vi "IO Docs.vi"(0 "Analog IO":dbl[](array[numeric]), 2 "BIAS DIFF":T3 {"DIFF" step=10.0; "BIAS" step=10.0}, 3 "Digital IO":bool[](array[boolean]), 4 "GXVALS Input":T1 {"g2rdggain" step=1e-05; "g2rdgoffset" step=1e-05; "g2spgain" step=1e-05; "g2spoffset" step=1e-05; "g1rdggain" step=1e-05; "g1rdgoffset" step=1e-05; "g1spgain" step=1e-05; "g1spoffset" step=1e-05}, 5 "Error In":errorcluster, 8 "User Creds":T2, 9 "OffsetGain":dbl[](array[numeric])) -> (10 "OffsetGain Out":dbl[](array[numeric]), 11 "BIAS DIFF Out":T3 {"DIFF" step=10.0; "BIAS" step=10.0}, 14 "Analog IO Out":dbl[](array[numeric]), 17 "GXVALS Output":T1 {"g2rdggain" step=1e-05; "g2rdgoffset" step=1e-05; "g2spgain" step=1e-05; "g2spoffset" step=1e-05; "g1rdggain" step=1e-05; "g1rdgoffset" step=1e-05; "g1spgain" step=1e-05; "g1spoffset" step=1e-05}, 19 "Error Out":errorcluster)   [LabVIEW 2023, in "QSM - IODocs.lvlib"]
uses:
  QSM - IODocs.lvlib
  Controls/AnalogIOAll.ctl
  Controls/AnalogIOsingle.ctl
  QSM - Main/Controls/biasdiff.ctl
  QSM - Main/Controls/gridvals.ctl
  UserCredentials.ctl
  Controls/State Machine Message.ctl
  Controls/Message Queue Element Position.ctl
  <vilib>/event_ctls.llb/usereventprio.ctl
  Controls/Event Handler Message.ctl
  QSM - Main/QSM - Main.lvlib
panel:
  in  "CLOSE":bool
  in  "GXVALS":T1 {"g2rdggain" step=1e-05; "g2rdgoffset" step=1e-05; "g2spgain" step=1e-05; "g2spoffset" step=1e-05; "g1rdggain" step=1e-05; "g1rdgoffset" step=1e-05; "g1spgain" step=1e-05; "g1spoffset" step=1e-05}
  out "DIO Cluster":T4
  in  "Analog IO Cluster":T5 {"AIO Cluster remIfrdg"."IOspgain" step=1e-05; "AIO Cluster remIfrdg"."IOspoffset" step=1e-05; "AIO Cluster remEfDrRdg"."IOspgain" step=1e-05; "AIO Cluster remEfDrRdg"."IOspoffset" step=1e-05; "AIO Cluster remEfDrSP"."IOspgain" step=1e-05; "AIO Cluster remEfDrSP"."IOspoffset" step=1e-05; "AIO Cluster remMArdg"."IOspgain" step=1e-05; "AIO Cluster remMArdg"."IOspoffset" step=1e-05; "AIO Cluster remMASP"."IOspgain" step=1e-05; "AIO Cluster remMASP"."IOspoffset" step=1e-05; "AIO Cluster remKVrdg"."IOspgain" step=1e-05; "AIO Cluster remKVrdg"."IOspoffset" step=1e-05; "AIO Cluster remKVSP"."IOspgain" step=1e-05; "AIO Cluster remKVSP"."IOspoffset" step=1e-05}
  # "ANALOG I/O"
  # "GRID TANK VALUES"
  # "DIGITAL I/O"
  # "OFFSET"
  # "OFFSET"
  # "GAIN"
  # "GAIN"
  # "OFFSET"
  # "OFFSET"
  # "GAIN"
  # "GAIN"
  # "OFFSET"
  # "OFFSET"
  # "GAIN"
  # "GAIN"
  # "OFFSET"
  # "OFFSET"
  # "GAIN"
  # "GAIN"
  # "OFFSET"
  # "OFFSET"
  # "GAIN"
  # "GAIN"
  # "OFFSET"
  # "OFFSET"
  # "GAIN"
  # "GAIN"
  # "remKVSP"
  # "remKVrdg"
  # "remMASP"
  # "remMArdg"
  # "remEfDrSP"
  # "remEfDrRdg"
  # "remIfrdg"
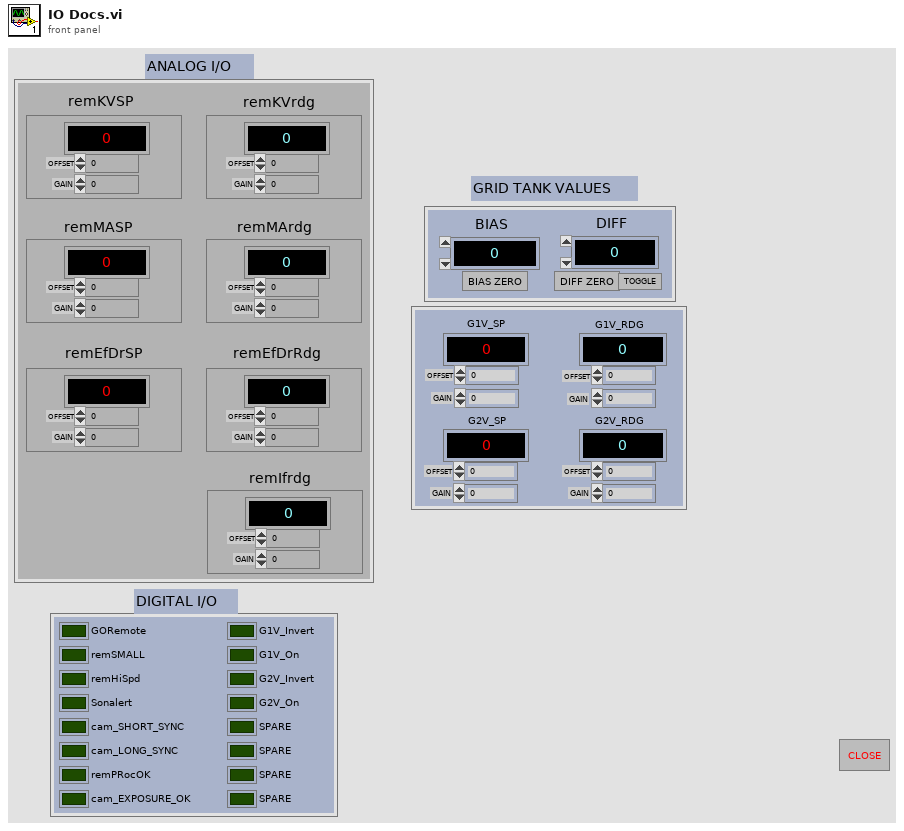
[diagram p1: front panel]
types:
  T1 = typedef "QSM - Main.lvlib/gridvals.ctl" = cluster{"G1V_SP":dbl, "G2V_SP":dbl, "G1V_RDG":dbl, "G2V_RDG":dbl, "g1spoffset":dbl, "g1spgain":dbl, "g1rdgoffset":dbl, "g1rdggain":dbl, "g2spoffset":dbl, "g2spgain":dbl, "g2rdgoffset":dbl, "g2rdggain":dbl}
  T2 = typedef "UserCredentials.ctl" = cluster{"Badge Number":string, "Name":string, "Access":enum16{"", "Operator", "Admin", "Engineer"}}
  T3 = typedef "QSM - Main.lvlib/biasdiff.ctl" = cluster{"BIAS":dbl, "BIAS_ZER":bool, "DIFF_ZER":bool, "DIFF_TOGGLE":bool, "DIFF":dbl}
  T4 = cluster{"GORemote":bool, "remSMALL":bool, "remHiSpd":bool, "Sonalert":bool, "cam_SHORT_SYNC":bool, "cam_LONG_SYNC":bool, "remPRocOK":bool, "cam_EXPOSURE_OK":bool, "G1V_Invert":bool, "G1V_On":bool, "G2V_Invert":bool, "G2V_On":bool, "SPARE":bool, "SPARE":bool, "SPARE":bool, "SPARE":bool}
  T5 = typedef "QSM - IODocs.lvlib/AnalogIOAll.ctl" = cluster{"AIO Cluster remKVSP":T6, "AIO Cluster remKVrdg":T6, "AIO Cluster remMASP":T6, "AIO Cluster remMArdg":T6, "AIO Cluster remEfDrSP":T6, "AIO Cluster remEfDrRdg":T6, "AIO Cluster remIfrdg":T6}
  T6 = typedef "QSM - IODocs.lvlib/AnalogIOsingle.ctl" = cluster{"I/O":dbl, "IOspoffset":dbl, "IOspgain":dbl}
  T7 = typedef "QSM - IODocs.lvlib/State Machine Message.ctl" = enum16{"Initialize", "BIAS ZERO", "DIFF ZERO", "DIFF TOGGLE", "UpdateAIO", "UpdateBiasDiff", "GxValsUpdate", "OffsetGainUpdate", "APIAIOUpdate", "APIGridValsUpdate", "APIBiasDiffUpdate", "Handle Error", "Exit"}
  T8 = typedef "QSM - IODocs.lvlib/User Event Reference.ctl" = refnum<user-event>
  T9 = typedef "QSM - IODocs.lvlib/User Event Registration Reference.ctl" = refnum<event-registration>
  T10 = typedef "QSM - IODocs.lvlib/Event Handler Message.ctl" = enum16{"Exit"}
  T11 = typedef "usereventprio.ctl" = enum32{"high priority", "normal priority"}
  T12 = cluster{"Value[0]":bool, "Value[1]":bool, "Value[2]":bool, "Value[3]":bool, "Value[4]":bool, "Value[5]":bool, "Value[6]":bool, "Value[7]":bool, "Value[8]":bool, "Value[9]":bool, "Value[10]":bool, "Value[11]":bool, "Value[12]":bool, "Value[13]":bool, "Value[14]":bool, "Value[15]":bool}
  T13 = cluster{"Value[0]":dbl, "Value[1]":dbl, "Value[2]":dbl, "Value[3]":dbl, "Value[4]":dbl, "Value[5]":dbl, "Value[6]":dbl, "Value[7]":dbl, "Value[8]":dbl, "Value[9]":dbl, "Value[10]":dbl, "Value[11]":dbl, "Value[12]":dbl, "Value[13]":dbl, "Value[14]":dbl, "Value[15]":dbl, "Value[16]":dbl, "Value[17]":dbl, "Value[18]":dbl, "Value[19]":dbl, "Value[20]":dbl, "Value[21]":dbl}
  T14 = enum8{"Enabled", "Disabled", "Disabled and Grayed Out"}
  T15 = cluster{"Value[0]":dbl, "Value[1]":dbl, "Value[2]":dbl, "Value[3]":dbl, "Value[4]":dbl, "Value[5]":dbl, "Value[6]":dbl, "Value[7]":dbl, "Value[8]":dbl, "Value[9]":dbl, "Value[10]":dbl}
  T16 = cluster{"Analog IO[0]":dbl, "Analog IO[1]":dbl, "Analog IO[2]":dbl, "Analog IO[3]":dbl, "Analog IO[4]":dbl, "Analog IO[5]":dbl, "Analog IO[6]":dbl, "Analog IO[7]":dbl, "Analog IO[8]":dbl, "Analog IO[9]":dbl, "Analog IO[10]":dbl}
  T17 = typedef "QSM - IODocs.lvlib/Message Queue Element Position.ctl" = enum16{"Front", "Back"}
  T18 = typedef "QMH - Library.lvlib/Event Handler Message.ctl" = enum16{"Exit"}
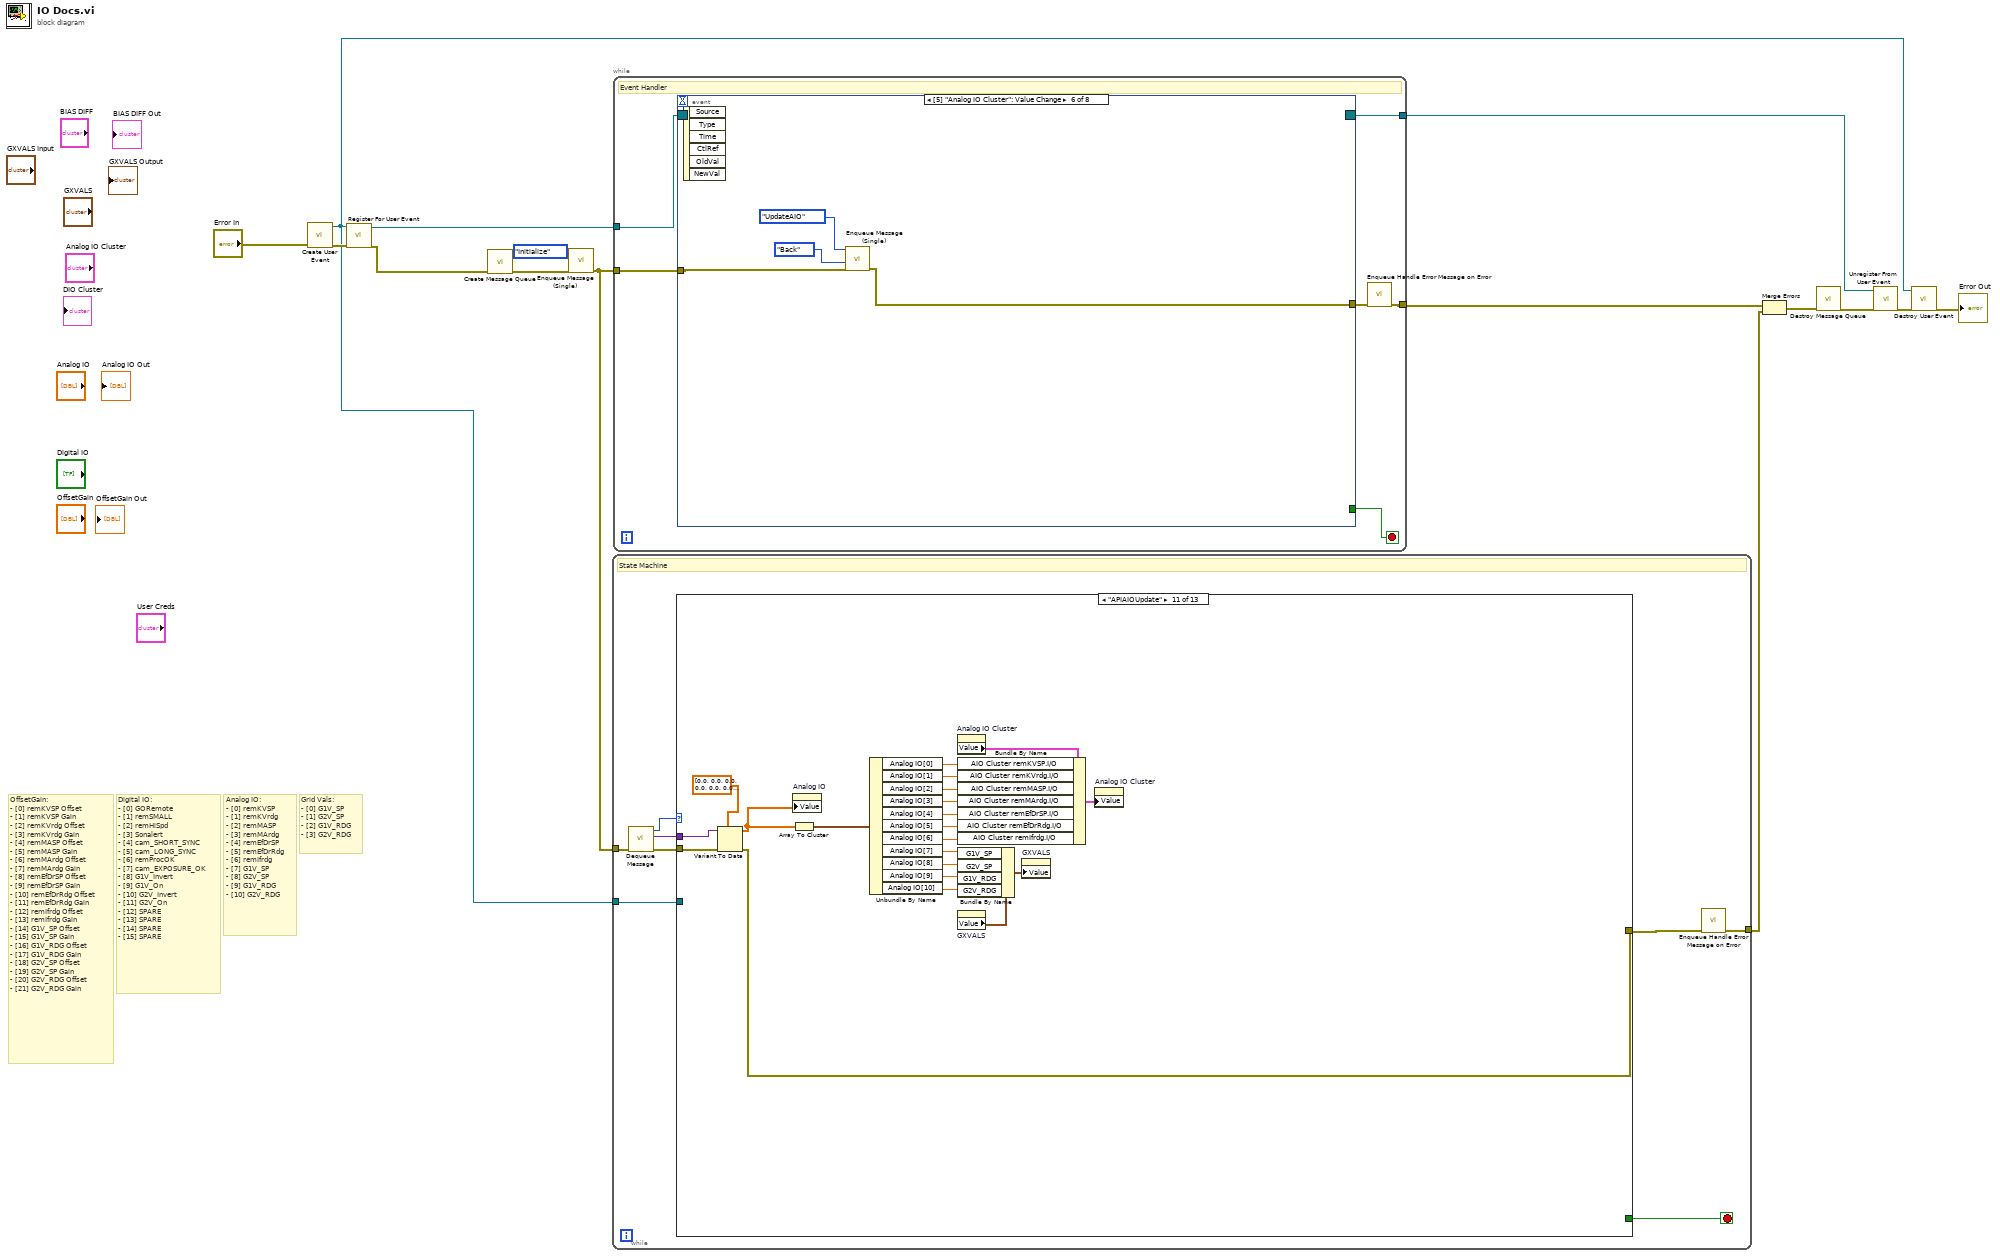
[diagram p0: block diagram]
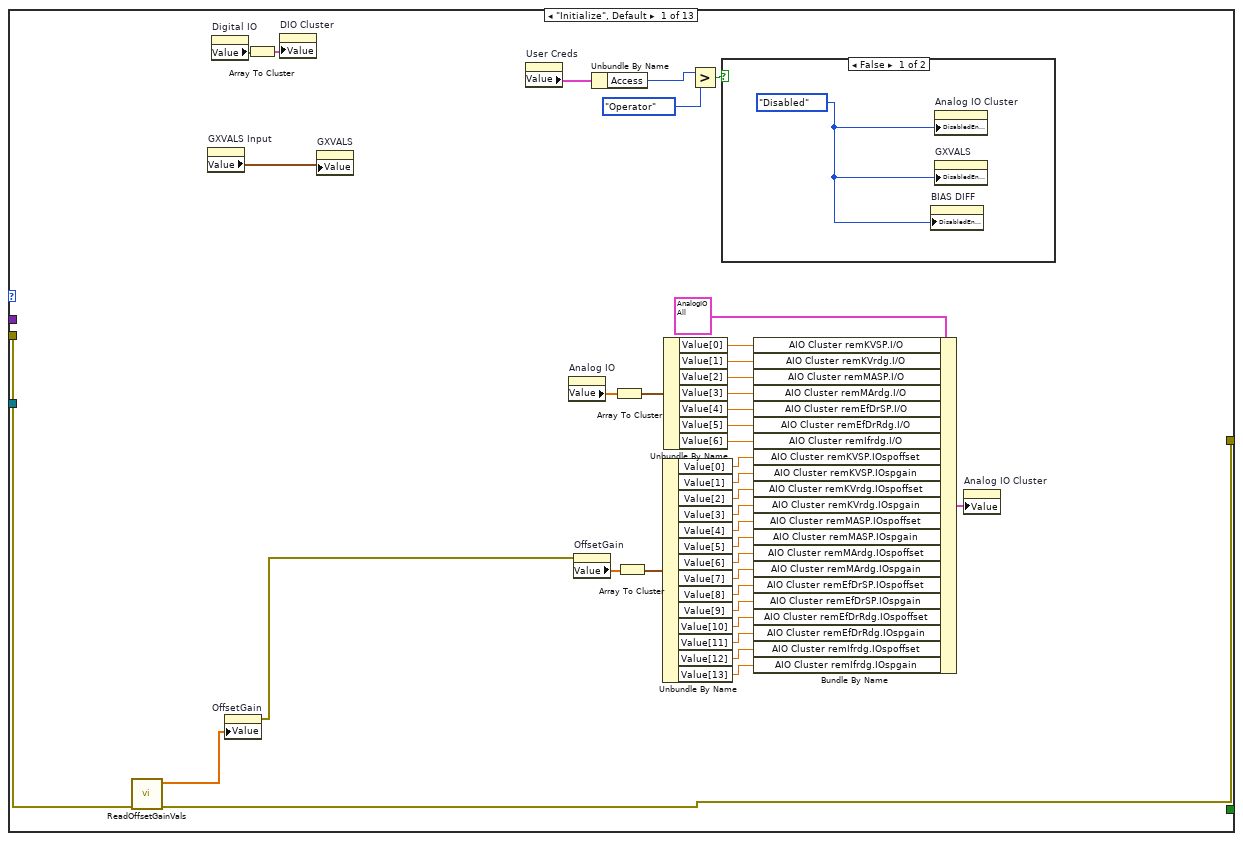
[diagram p2: hidden frame]
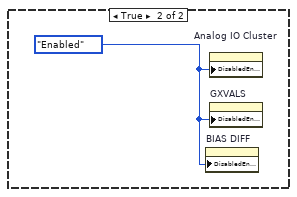
[diagram p3: hidden frame]
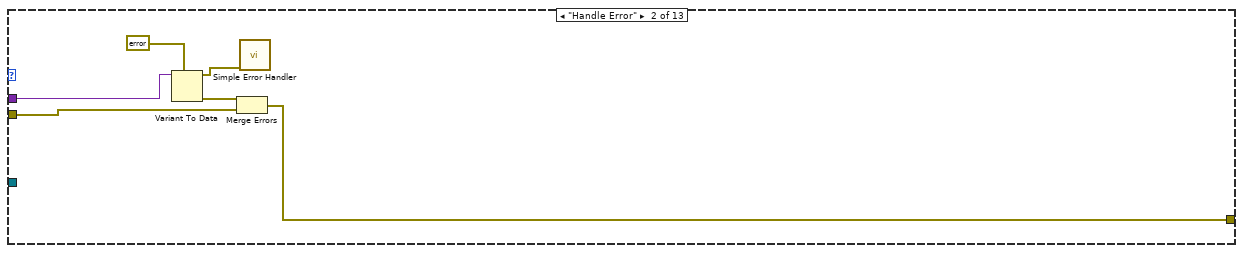
[diagram p4: hidden frame]
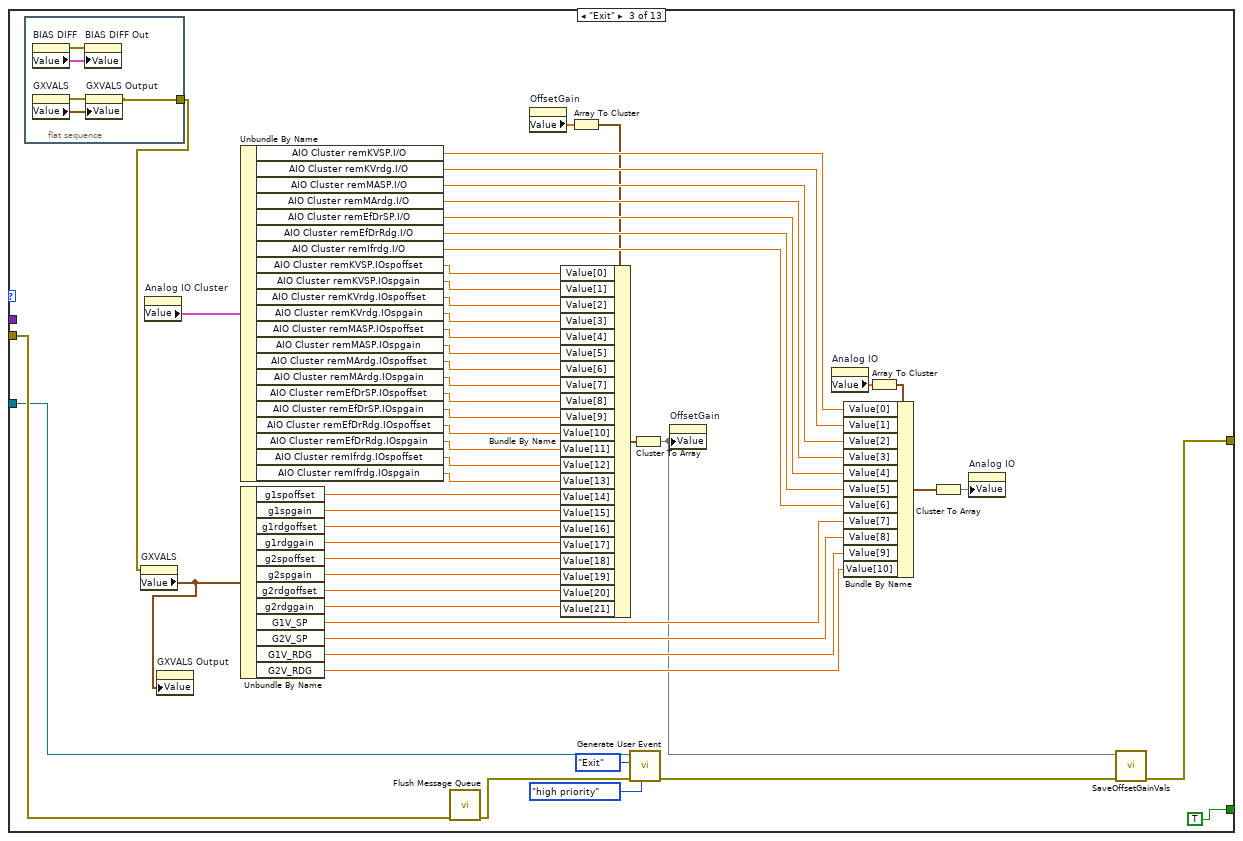
[diagram p5: hidden frame]
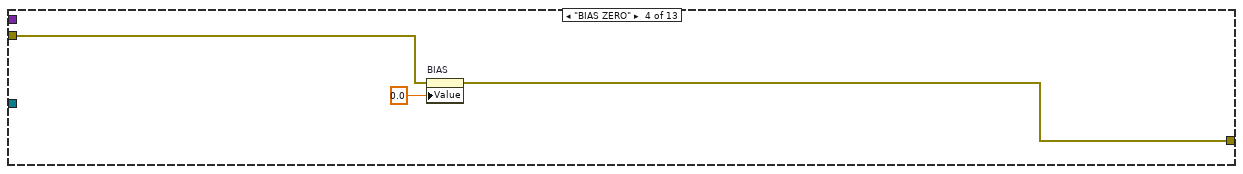
[diagram p6: hidden frame]
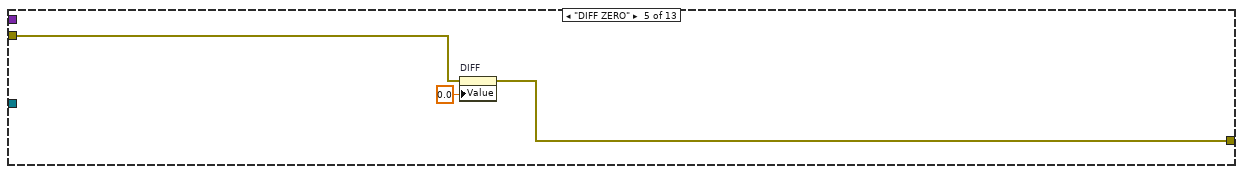
[diagram p7: hidden frame]
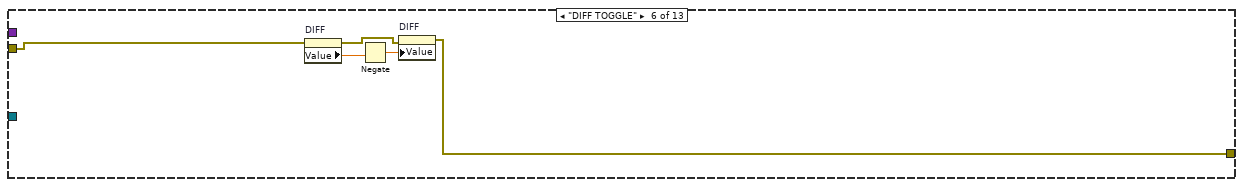
[diagram p8: hidden frame]
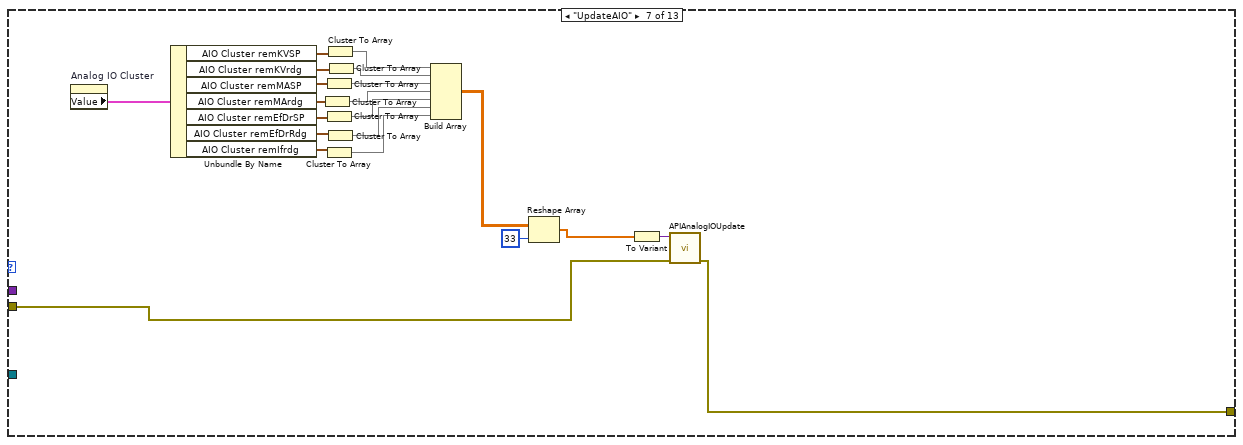
[diagram p9: hidden frame]
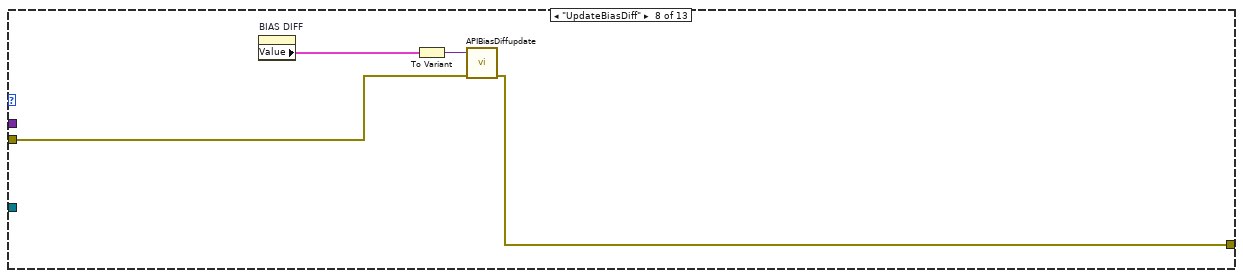
[diagram p10: hidden frame]
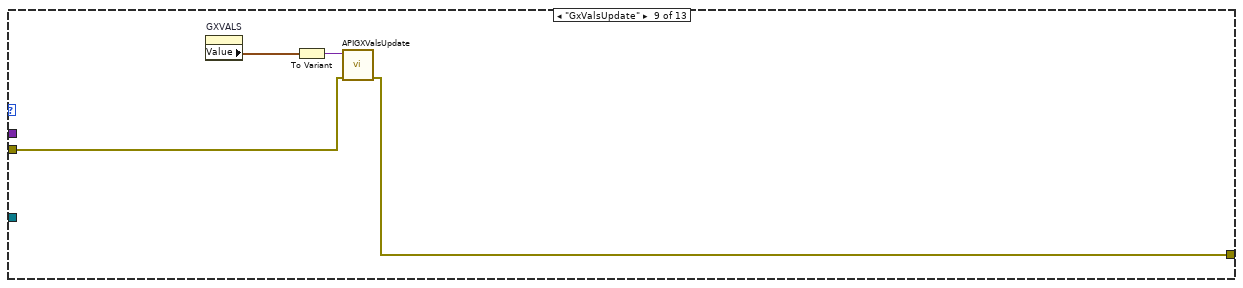
[diagram p11: hidden frame]
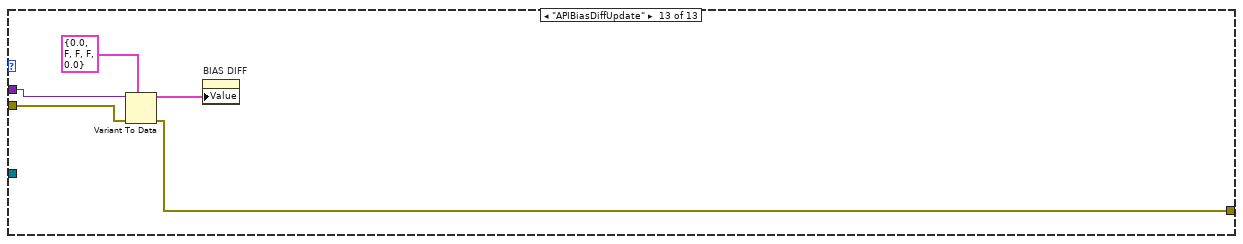
[diagram p14: hidden frame]
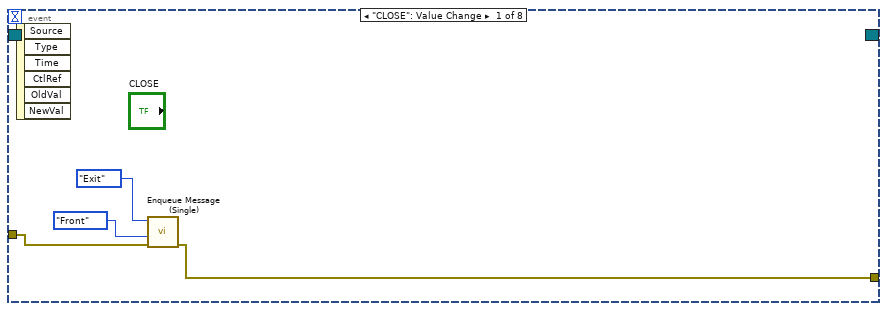
[diagram p15: hidden frame]
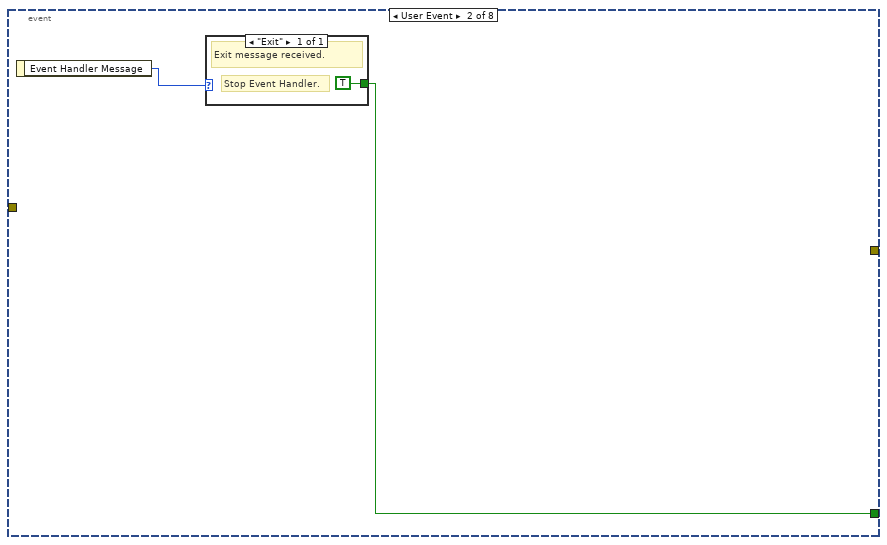
[diagram p16: hidden frame]
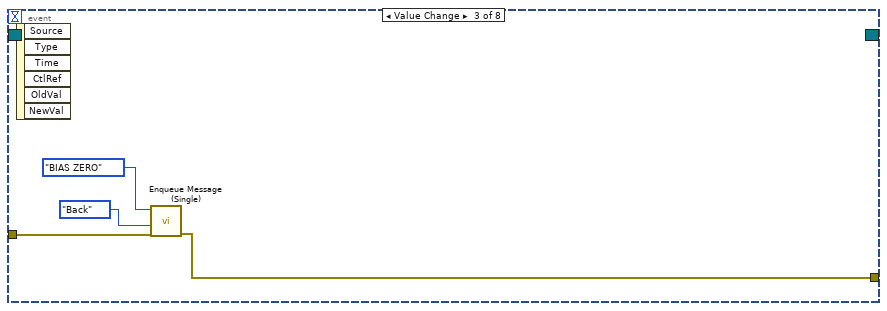
[diagram p17: hidden frame]
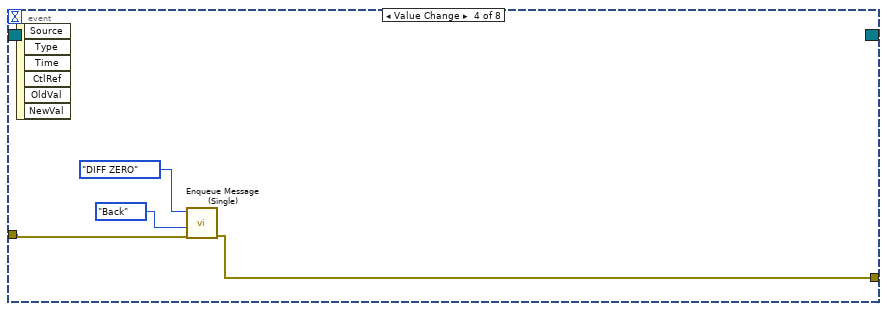
[diagram p18: hidden frame]
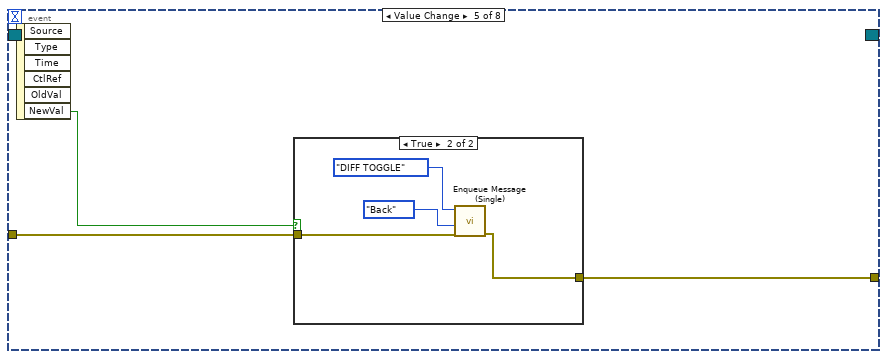
[diagram p19: hidden frame]
diagram:
  # "OffsetGain:\n- [0] remKVSP Offset\n- [1] remKVSP Gain\n- [2] remKVrdg Offset\n- [3] remKVrdg Gain\n- [4] remMASP Offset\n- [5] remMASP Gain\n- [6] remMArdg Offset\n- [7] remMArdg Gain\n- [8] remEfDrSP Offset\n- [9] remEfDrSP Gain\n- [10] remEfDrRdg Offset\n- [11] remEfDrRdg Gain\n- [12] remIfrdg Offset\n- [13] remIfrdg Gain\n- [14] G1V_SP Offset\n- [15] G1V_SP Gain\n- [16] G1V_RDG Offset\n- [17] G1V_RDG Gain\n- [18] G2V_SP Offset\n- [19] G2V_SP Gain\n- [20] G2V_RDG Offset\n- [21] G2V_RDG Gain"
  # "Digital IO:\n- [0] GORemote\n- [1] remSMALL\n- [2] remHiSpd\n- [3] Sonalert\n- [4] cam_SHORT_SYNC\n- [5] cam_LONG_SYNC\n- [6] remProcOK\n- [7] cam_EXPOSURE_OK\n- [8] G1V_Invert\n- [9] G1V_On\n- [10] G2V_Invert\n- [11] G2V_On\n- [12] SPARE\n- [13] SPARE\n- [14] SPARE\n- [15] SPARE"
  # "Grid Vals:\n- [0] G1V_SP\n- [1] G2V_SP\n- [2] G1V_RDG\n- [3] G2V_RDG"
  # "Analog IO:\n- [0] remKVSP\n- [1] remKVrdg\n- [2] remMASP\n- [3] remMArdg\n- [4] remEfDrSP\n- [5] remEfDrRdg\n- [6] remIfrdg\n- [7] G1V_SP\n- [8] G2V_SP\n- [9] G1V_RDG\n- [10] G2V_RDG"
  n1 = call "Create User Event.vi"("Error In"="Error In") -> ("Error Out"=w8:errorcluster, "User Event Reference"=w1:T8)  [unwired: 9 in]
  n2 = call "Register For User Event.vi"("Error In"=w8, "User Event Reference"=w1) -> ("Error Out"=w7:errorcluster, "User Event Registration Reference"=w6:T9)  [unwired: 8 in]
  n3 = call "Create Message Queue.vi"("Error In"=w7) -> ("Error Out"=w15:errorcluster)  [unwired: 10 in]
  n4 = call "Enqueue Message (Single).vi"("Error In"=w15, "State Machine Message"=State_Machine_Message."Initialize") -> ("Error Out"=w10:errorcluster)  [unwired: 9 in]
  n5 = while {
    tunnel: [w22] -> w13
    tunnel: w10 -> [w17]
    tunnel: w1 -> [w16]
    stop <- w23 stop-if-true
    # "State Machine"
    n6 = call "Dequeue Message.vi"("Error In"=w17) -> ("Error Out"=w21:errorcluster, "Data"=w19:variant, "State Machine Message"=w20:T7)  [unwired: 8 in]
    n7 = case shown="\"APIAIOUpdate\"" w20 {
      tunnel: [_ _ TRUE _ _ _ _ _ _ _ _ _ _] -> w23
      tunnel: w21 -> [w27 w66 w121 w127 w130 w136 w157 w161 w165 w167 w187 w189 w192]
      tunnel: w19 -> [_ w65 _ _ _ _ _ _ _ _ w188 _ w194]
      tunnel: [w26 w64 w71 w129 w132 w133 w156 w160 w164 w167 w186 w189 w191] -> w18
      tunnel: w16 -> [_ _ w73 _ _ _ _ _ _ _ _ _ _]
      frame "Initialize", Default {
        n8 = call "ReadOffsetGainVals.vi"("error in"=w27) -> ("error out"=w26:errorcluster, "Array"=w25:dbl[])  [unwired: 9 in]
        n9 = property on="GXVALS Input" class="Clust (strict)"() -> ("Value"=w28:T1)  [unwired: 2 in, 2 out]
        n10 = property on="Digital IO" class="Arr (strict)"() -> ("Value"=w58:bool[])  [unwired: 2 in, 2 out]
        n11 = property on="OffsetGain" class="Arr (strict)"("Value"=w25) -> (error out=w24:errorcluster)  [unwired: 2 in, 1 out]
        n12 = Array To Cluster(array=w58) -> (cluster=w57:T12)
        n13 = property on="DIO Cluster" class="Clust (strict)"("Value"=w57) -> ()  [unwired: 2 in, 2 out]
        n14 = property on="GXVALS" class="Clust (strict)"("Value"=w28) -> ()  [unwired: 2 in, 2 out]
        n15 = property on="User Creds" class="Clust (strict)"() -> ("Value"=w31:T2)  [unwired: 2 in, 2 out]
        n16 = property on="Analog IO" class="Arr (strict)"() -> ("Value"=w61:dbl[])  [unwired: 2 in, 2 out]
        n17 = property on="OffsetGain" class="Arr (strict)"(error in=w24) -> ("Value"=w49:dbl[])  [unwired: 1 in, 2 out]
        n18 = Unbundle By Name(w31) -> ("Access"=w30:enum16{"", "Operator", "Admin", "Engineer"})
        n19 = Array To Cluster(array=w61) -> (cluster=w33:T13)
        n20 = Array To Cluster(array=w49) -> (cluster=w48:T13)
        n21 = Unbundle By Name(w48) -> ("Value[0]"=w47:dbl, "Value[1]"=w46:dbl, "Value[2]"=w45:dbl, "Value[3]"=w44:dbl, "Value[4]"=w43:dbl, "Value[5]"=w42:dbl, "Value[6]"=w41:dbl, "Value[7]"=w40:dbl, "Value[8]"=w39:dbl, "Value[9]"=w38:dbl, "Value[10]"=w37:dbl, "Value[11]"=w36:dbl, "Value[12]"=w35:dbl, "Value[13]"=w34:dbl)
        n22 = Unbundle By Name(w33) -> ("Value[0]"=w56:dbl, "Value[1]"=w55:dbl, "Value[2]"=w54:dbl, "Value[3]"=w53:dbl, "Value[4]"=w52:dbl, "Value[5]"=w51:dbl, "Value[6]"=w50:dbl)
        n23 = Greater?(x=w30, y=enum16{"", "Operator", "Admin", "Engineer"}."Operator") -> (0:w32:bool)
        n24 = case shown="False" w32 {
          frame False {
            w62 = T14."Disabled" ("Disabled")
            n25 = property on="BIAS DIFF" class="Clust (strict)"("DisabledEnum"=w62) -> ()  [unwired: 2 in, 2 out]
            n26 = property on="Analog IO Cluster" class="Clust (strict)"("DisabledEnum"=w62) -> ()  [unwired: 2 in, 2 out]
            n27 = property on="GXVALS" class="Clust (strict)"("DisabledEnum"=w62) -> ()  [unwired: 2 in, 2 out]
          }
          frame True {
            w63 = T14."Enabled" ("Disabled")
            n28 = property on="BIAS DIFF" class="Clust (strict)"("DisabledEnum"=w63) -> ()  [unwired: 2 in, 2 out]
            n29 = property on="Analog IO Cluster" class="Clust (strict)"("DisabledEnum"=w63) -> ()  [unwired: 2 in, 2 out]
            n30 = property on="GXVALS" class="Clust (strict)"("DisabledEnum"=w63) -> ()  [unwired: 2 in, 2 out]
          }
        }
        n31 = Bundle By Name(cluster=T5 {"AIO Cluster remKVSP"={"I/O"=0.0, "IOspoffset"=0.0, "IOspgain"=0.0}, "AIO Cluster remKVrdg"={"I/O"=0.0, "IOspoffset"=0.0, "IOspgain"=0.0}, "AIO Cluster remMASP"={"I/O"=0.0, "IOspoffset"=0.0, "IOspgain"=0.0}, "AIO Cluster remMArdg"={"I/O"=0.0, "IOspoffset"=0.0, "IOspgain"=0.0}, "AIO Cluster remEfDrSP"={"I/O"=0.0, "IOspoffset"=0.0, "IOspgain"=0.0}, "AIO Cluster remEfDrRdg"={"I/O"=0.0, "IOspoffset"=0.0, "IOspgain"=0.0}, "AIO Cluster remIfrdg"={"I/O"=0.0, "IOspoffset"=0.0, "IOspgain"=0.0}} ("Analog IO Cluster"), "AIO Cluster remKVSP.I/O"=w56, "AIO Cluster remKVrdg.I/O"=w55, "AIO Cluster remMASP.I/O"=w54, "AIO Cluster remMArdg.I/O"=w53, "AIO Cluster remEfDrSP.I/O"=w52, "AIO Cluster remEfDrRdg.I/O"=w51, "AIO Cluster remIfrdg.I/O"=w50, "AIO Cluster remKVSP.IOspoffset"=w47, "AIO Cluster remKVSP.IOspgain"=w46, "AIO Cluster remKVrdg.IOspoffset"=w45, "AIO Cluster remKVrdg.IOspgain"=w44, "AIO Cluster remMASP.IOspoffset"=w43, "AIO Cluster remMASP.IOspgain"=w42, "AIO Cluster remMArdg.IOspoffset"=w41, "AIO Cluster remMArdg.IOspgain"=w40, "AIO Cluster remEfDrSP.IOspoffset"=w39, "AIO Cluster remEfDrSP.IOspgain"=w38, "AIO Cluster remEfDrRdg.IOspoffset"=w37, "AIO Cluster remEfDrRdg.IOspgain"=w36, "AIO Cluster remIfrdg.IOspoffset"=w35, "AIO Cluster remIfrdg.IOspgain"=w34) -> (w60:T5)
        n32 = property on="Analog IO Cluster" class="Clust (strict)"("Value"=w60) -> ()  [unwired: 2 in, 2 out]
      }
      frame "Handle Error" {
        n33 = Variant To Data(type=errorcluster {"status"=FALSE, "code"=0, "source"=""} ("Error In"), Variant=w65) -> (data=w67:errorcluster, error out=w68:errorcluster)  [unwired: 1 in]
        n34 = Merge Errors(w68, w66) -> (w64:errorcluster)
        n35 = call <vilib>:"Simple Error Handler.vi"("error in (no error)"=w67) -> ()  [unwired: 4 in, 5 out]
      }
      frame "Exit" {
        n36 = flat-sequence {
          tunnel: [w122] -> w96
          frame #0 {
            n37 = property on="BIAS DIFF" class="Clust (strict)"() -> (error out=w126:errorcluster, "Value"=w125:T3)  [unwired: 2 in, 1 out]
            n38 = property on="GXVALS" class="Clust (strict)"() -> (error out=w124:errorcluster, "Value"=w123:T1)  [unwired: 2 in, 1 out]
            n39 = property on="BIAS DIFF Out" class="Clust (strict)"(error in=w126, "Value"=w125) -> ()  [unwired: 1 in, 2 out]
            n40 = property on="GXVALS Output" class="Clust (strict)"(error in=w124, "Value"=w123) -> (error out=w122:errorcluster)  [unwired: 1 in, 1 out]
          }
        }
        n41 = property on="GXVALS" class="Clust (strict)"(error in=w96) -> ("Value"=w77:T1)  [unwired: 1 in, 2 out]
        n42 = property on="Analog IO Cluster" class="Clust (strict)"() -> ("Value"=w119:T5)  [unwired: 2 in, 2 out]
        n43 = property on="GXVALS Output" class="Clust (strict)"("Value"=w77) -> ()  [unwired: 2 in, 2 out]
        n44 = Unbundle By Name(w119) -> ("AIO Cluster remKVSP.I/O"=w95:dbl, "AIO Cluster remKVrdg.I/O"=w94:dbl, "AIO Cluster remMASP.I/O"=w93:dbl, "AIO Cluster remMArdg.I/O"=w92:dbl, "AIO Cluster remEfDrSP.I/O"=w91:dbl, "AIO Cluster remEfDrRdg.I/O"=w90:dbl, "AIO Cluster remIfrdg.I/O"=w89:dbl, "AIO Cluster remKVSP.IOspoffset"=w118:dbl, "AIO Cluster remKVSP.IOspgain"=w117:dbl, "AIO Cluster remKVrdg.IOspoffset"=w116:dbl, "AIO Cluster remKVrdg.IOspgain"=w115:dbl, "AIO Cluster remMASP.IOspoffset"=w114:dbl, "AIO Cluster remMASP.IOspgain"=w113:dbl, "AIO Cluster remMArdg.IOspoffset"=w112:dbl, "AIO Cluster remMArdg.IOspgain"=w111:dbl, "AIO Cluster remEfDrSP.IOspoffset"=w110:dbl, "AIO Cluster remEfDrSP.IOspgain"=w109:dbl, "AIO Cluster remEfDrRdg.IOspoffset"=w108:dbl, "AIO Cluster remEfDrRdg.IOspgain"=w107:dbl, "AIO Cluster remIfrdg.IOspoffset"=w106:dbl, "AIO Cluster remIfrdg.IOspgain"=w105:dbl)
        n45 = Unbundle By Name(w77) -> ("g1spoffset"=w85:dbl, "g1spgain"=w84:dbl, "g1rdgoffset"=w83:dbl, "g1rdggain"=w82:dbl, "g2spoffset"=w81:dbl, "g2spgain"=w80:dbl, "g2rdgoffset"=w79:dbl, "g2rdggain"=w78:dbl, "G1V_SP"=w104:dbl, "G2V_SP"=w103:dbl, "G1V_RDG"=w102:dbl, "G2V_RDG"=w101:dbl)
        n46 = call "Flush Message Queue.vi"("Error In"=w121) -> ("Error Out"=w76:errorcluster)  [unwired: 9 in, 1 out]
        n47 = property on="OffsetGain" class="Arr (strict)"() -> ("Value"=w88:dbl[])  [unwired: 2 in, 2 out]
        n48 = Array To Cluster(array=w88) -> (cluster=w86:T13)
        n49 = Bundle By Name(cluster=w86, "Value[0]"=w118, "Value[1]"=w117, "Value[2]"=w116, "Value[3]"=w115, "Value[4]"=w114, "Value[5]"=w113, "Value[6]"=w112, "Value[7]"=w111, "Value[8]"=w110, "Value[9]"=w109, "Value[10]"=w108, "Value[11]"=w107, "Value[12]"=w106, "Value[13]"=w105, "Value[14]"=w85, "Value[15]"=w84, "Value[16]"=w83, "Value[17]"=w82, "Value[18]"=w81, "Value[19]"=w80, "Value[20]"=w79, "Value[21]"=w78) -> (w87:T13)
        n50 = call "Generate User Event.vi"("User Event Priority"=usereventprio."high priority", "Error In"=w76, "Event Handler Message"=Event_Handler_Message."Exit", "User Event Reference"=w73) -> ("Error Out"=w72:errorcluster)  [unwired: 7 in]
        n51 = Cluster To Array(cluster=w87) -> (array=w70:dbl[])
        n52 = property on="OffsetGain" class="Arr (strict)"("Value"=w70) -> ()  [unwired: 2 in, 2 out]
        n53 = property on="Analog IO" class="Arr (strict)"() -> ("Value"=w98:dbl[])  [unwired: 2 in, 2 out]
        n54 = Array To Cluster(array=w98) -> (cluster=w99:T15)
        n55 = Bundle By Name(cluster=w99, "Value[0]"=w95, "Value[1]"=w94, "Value[2]"=w93, "Value[3]"=w92, "Value[4]"=w91, "Value[5]"=w90, "Value[6]"=w89, "Value[7]"=w104, "Value[8]"=w103, "Value[9]"=w102, "Value[10]"=w101) -> (w100:T15)
        n56 = Cluster To Array(cluster=w100) -> (array=w97:dbl[])
        n57 = property on="Analog IO" class="Arr (strict)"("Value"=w97) -> ()  [unwired: 2 in, 2 out]
        n58 = call "SaveOffsetGainVals.vi"("error in"=w72, "OffsetGain Array"=w70) -> ("error out"=w71:errorcluster)  [unwired: 9 in]
      }
      frame "BIAS ZERO" {
        n59 = property on="BIAS" class="DigNum (strict)"(error in=w127, "Value"=0.0 ("BIAS")) -> (error out=w129:errorcluster)  [unwired: 1 in, 1 out]
      }
      frame "DIFF ZERO" {
        n60 = property on="DIFF" class="DigNum (strict)"(error in=w130, "Value"=0.0 ("BIAS")) -> (error out=w132:errorcluster)  [unwired: 1 in, 1 out]
      }
      frame "DIFF TOGGLE" {
        n61 = property on="DIFF" class="DigNum (strict)"(error in=w136) -> (error out=w134:errorcluster, "Value"=w135:dbl)  [unwired: 1 in, 1 out]
        n62 = Negate(x=w135) -> (-x=w137:dbl)
        n63 = property on="DIFF" class="DigNum (strict)"(error in=w134, "Value"=w137) -> (error out=w133:errorcluster)  [unwired: 1 in, 1 out]
      }
      frame "UpdateAIO" {
        n64 = property on="Analog IO Cluster" class="Clust (strict)"() -> ("Value"=w155:T5)  [unwired: 2 in, 2 out]
        n65 = Unbundle By Name(w155) -> ("AIO Cluster remKVSP"=w154:T6, "AIO Cluster remKVrdg"=w153:T6, "AIO Cluster remMASP"=w152:T6, "AIO Cluster remMArdg"=w151:T6, "AIO Cluster remEfDrSP"=w150:T6, "AIO Cluster remEfDrRdg"=w149:T6, "AIO Cluster remIfrdg"=w148:T6)
        n66 = Cluster To Array(cluster=w151) -> (array=w144:dbl[])
        n67 = Cluster To Array(cluster=w152) -> (array=w145:dbl[])
        n68 = Cluster To Array(cluster=w150) -> (array=w143:dbl[])
        n69 = Cluster To Array(cluster=w148) -> (array=w141:dbl[])
        n70 = Cluster To Array(cluster=w154) -> (array=w147:dbl[])
        n71 = Cluster To Array(cluster=w149) -> (array=w142:dbl[])
        n72 = Cluster To Array(cluster=w153) -> (array=w146:dbl[])
        n73 = Build Array(w147, w146, w145, w144, w143, w142, w141) -> (w140:dbl[][])
        n74 = Reshape Array(w140, 33 ("dimension size")) -> (w138:dbl[])
        n75 = To Variant(anything=w138) -> (Variant=w158:variant)
        n76 = call "APIAnalogIOUpdate.vi"("Error In"=w157, "Data"=w158) -> ("Error Out"=w156:errorcluster)  [unwired: 9 in]
      }
      frame "UpdateBiasDiff" {
        n77 = property on="BIAS DIFF" class="Clust (strict)"() -> ("Value"=w159:T3)  [unwired: 2 in, 2 out]
        n78 = To Variant(anything=w159) -> (Variant=w162:variant)
        n79 = call "APIBiasDiffupdate.vi"("Error In"=w161, "Data"=w162) -> ("Error Out"=w160:errorcluster)  [unwired: 9 in]
      }
      frame "GxValsUpdate" {
        n80 = property on="GXVALS" class="Clust (strict)"() -> ("Value"=w163:T1)  [unwired: 2 in, 2 out]
        n81 = To Variant(anything=w163) -> (Variant=w166:variant)
        n82 = call "APIGXValsUpdate.vi"("Error In"=w165, "Data"=w166) -> ("Error Out"=w164:errorcluster)  [unwired: 9 in]
      }
      frame "OffsetGainUpdate" {
      }
      frame "APIAIOUpdate" {
        n83 = Variant To Data(error in=w187, type=dbl[] [0.0, 0.0, 0.0, 0.0, 0.0, 0.0, 0.0, 0.0, 0.0, 0.0, 0.0] ("Analog IO"), Variant=w188) -> (data=w184:dbl[], error out=w186:errorcluster)
        n84 = Array To Cluster(array=w184) -> (cluster=w183:T16)
        n85 = property on="Analog IO" class="Arr (strict)"("Value"=w184) -> ()  [unwired: 2 in, 2 out]
        n86 = Unbundle By Name(w183) -> ("Analog IO[0]"=w180:dbl, "Analog IO[1]"=w179:dbl, "Analog IO[2]"=w178:dbl, "Analog IO[3]"=w177:dbl, "Analog IO[4]"=w176:dbl, "Analog IO[5]"=w175:dbl, "Analog IO[6]"=w174:dbl, "Analog IO[7]"=w171:dbl, "Analog IO[8]"=w170:dbl, "Analog IO[9]"=w169:dbl, "Analog IO[10]"=w168:dbl)
        n87 = property on="Analog IO Cluster" class="Clust (strict)"() -> ("Value"=w182:T5)  [unwired: 2 in, 2 out]
        n88 = Bundle By Name(cluster=w182, "AIO Cluster remKVSP.I/O"=w180, "AIO Cluster remKVrdg.I/O"=w179, "AIO Cluster remMASP.I/O"=w178, "AIO Cluster remMArdg.I/O"=w177, "AIO Cluster remEfDrSP.I/O"=w176, "AIO Cluster remEfDrRdg.I/O"=w175, "AIO Cluster remIfrdg.I/O"=w174) -> (w181:T5)
        n89 = property on="GXVALS" class="Clust (strict)"() -> ("Value"=w173:T1)  [unwired: 2 in, 2 out]
        n90 = Bundle By Name(cluster=w173, "G1V_SP"=w171, "G2V_SP"=w170, "G1V_RDG"=w169, "G2V_RDG"=w168) -> (w172:T1)
        n91 = property on="GXVALS" class="Clust (strict)"("Value"=w172) -> ()  [unwired: 2 in, 2 out]
        n92 = property on="Analog IO Cluster" class="Clust (strict)"("Value"=w181) -> ()  [unwired: 2 in, 2 out]
      }
      frame "APIGridValsUpdate" {
      }
      frame "APIBiasDiffUpdate" {
        n93 = Variant To Data(error in=w192, type=T3 {"BIAS"=0.0, "BIAS_ZER"=FALSE, "DIFF_ZER"=FALSE, "DIFF_TOGGLE"=FALSE, "DIFF"=0.0} ("BIAS DIFF"), Variant=w194) -> (data=w190:T3, error out=w191:errorcluster)
        n94 = property on="BIAS DIFF" class="Clust (strict)"("Value"=w190) -> ()  [unwired: 2 in, 2 out]
      }
    }
    n95 = call "Enqueue Handle Error Message on Error.vi"("Error In"=w18) -> ("Error Out"=w22:errorcluster)  [unwired: 10 in]
  }
  n96 = while {
    tunnel: w10 -> [w199]
    tunnel: [w198] -> w11
    tunnel: w6 -> [w196]
    tunnel: [w195] -> w2
    stop <- w200 stop-if-true
    # "Event Handler"
    n97 = event shown="[5] \"Analog IO Cluster\": Value Change" {
      selector: w196 -> [_ _ _ _ _ _ _ _]
      dyn-events: [_ _ _ _ _ _ _ _] -> w195
      timeout: _ -> [_ _ _ _ _ _ _ _]
      tunnel: [_ w205 _ _ _ _ _ _] -> w200
      tunnel: w199 -> [w203 _ w209 w213 w218 w225 w229 w233]
      tunnel: [w201 _ w208 w212 w217 w224 w228 w232] -> w197
      event "CLOSE": Value Change {
        n98 = event-data() -> ()  [unwired: 1 in, 6 out]
        n99 = call "Enqueue Message (Single).vi"("Error In"=w203, "Message Position"=Message_Queue_Element_Position."Front", "State Machine Message"=State_Machine_Message."Exit") -> ("Error Out"=w201:errorcluster)  [unwired: 8 in]
      }
      event User Event {
        n100 = event-data() -> ("Event Handler Message"=w206:T18)  [unwired: 1 in]
        n101 = case shown="\"Exit\"" w206 {
          tunnel: [TRUE] -> w205
          frame "Exit" {
            # "Stop Event Handler."
            # "Exit message received."
          }
        }
      }
      event Value Change {
        n102 = event-data() -> ()  [unwired: 1 in, 6 out]
        n103 = call "Enqueue Message (Single).vi"("Error In"=w209, "Message Position"=Message_Queue_Element_Position."Back", "State Machine Message"=State_Machine_Message."BIAS ZERO") -> ("Error Out"=w208:errorcluster)  [unwired: 8 in]
      }
      event Value Change {
        n104 = event-data() -> ()  [unwired: 1 in, 6 out]
        n105 = call "Enqueue Message (Single).vi"("Error In"=w213, "Message Position"=Message_Queue_Element_Position."Back", "State Machine Message"=State_Machine_Message."DIFF ZERO") -> ("Error Out"=w212:errorcluster)  [unwired: 8 in]
      }
      event Value Change {
        n106 = event-data() -> ("NewVal"=w216:bool)  [unwired: 1 in, 5 out]
        n107 = case shown="True" w216 {
          tunnel: w218 -> [w219 w221]
          tunnel: [w219 w220] -> w217
          frame False {
          }
          frame True {
            n108 = call "Enqueue Message (Single).vi"("Error In"=w221, "Message Position"=Message_Queue_Element_Position."Back", "State Machine Message"=State_Machine_Message."DIFF TOGGLE") -> ("Error Out"=w220:errorcluster)  [unwired: 8 in]
          }
        }
      }
      event Value Change {
        n109 = event-data() -> ()  [unwired: 1 in, 6 out]
        n110 = call "Enqueue Message (Single).vi"("Error In"=w225, "Message Position"=Message_Queue_Element_Position."Back", "State Machine Message"=State_Machine_Message."UpdateAIO") -> ("Error Out"=w224:errorcluster)  [unwired: 8 in]
      }
      event Value Change {
        n111 = event-data() -> ()  [unwired: 1 in, 6 out]
        n112 = call "Enqueue Message (Single).vi"("Error In"=w229, "Message Position"=Message_Queue_Element_Position."Back", "State Machine Message"=State_Machine_Message."GxValsUpdate") -> ("Error Out"=w228:errorcluster)  [unwired: 8 in]
      }
      event Value Change {
        n113 = event-data() -> ()  [unwired: 1 in, 6 out]
        n114 = call "Enqueue Message (Single).vi"("Error In"=w233, "Message Position"=Message_Queue_Element_Position."Back", "State Machine Message"=State_Machine_Message."UpdateBiasDiff") -> ("Error Out"=w232:errorcluster)  [unwired: 8 in]
      }
    }
    n115 = call "Enqueue Handle Error Message on Error.vi"("Error In"=w197) -> ("Error Out"=w198:errorcluster)  [unwired: 10 in]
  }
  n116 = Merge Errors(w11, w13) -> (w12:errorcluster)
  n117 = call "Destroy Message Queue.vi"("Error In"=w12) -> ("Error Out"=w4:errorcluster)  [unwired: 10 in]
  n118 = call "Unregister From User Event.vi"("Error In"=w4, "User Event Registration Reference"=w2) -> ("Error Out"=w5:errorcluster)  [unwired: 9 in]
  n119 = call "Destroy User Event.vi"("Error In"=w5, "User Event Reference"=w1) -> ("Error Out"=→"Error Out":errorcluster)  [unwired: 9 in]
